vi "Agilent 3446X Series Acquire Multiple.vi"() -> ()   [LabVIEW 2021]
doc: "This example shows how to configure a measurement and take multiple readings."
uses:
  <instrlib>/Agilent 3446X Series/Public/Data/Read (Multiple Points).vi
  <instrlib>/Agilent 3446X Series/Agilent 3446X Series.lvlib
panel:
  in  "error in":errorcluster
  out "error out":errorcluster
  in  "Timeout(s)":i32=10000 format="%#.6g"
  in  "Sample Count":i32=1
  in  "Measurement Function":i32(ring)=10 items=["Continuity", "Current AC", "Current DC", "Diode", "Frequency", "Resistance 4-wire", "Period", "Resistance 2-wire", "Temperature", "Voltage AC", "Voltage DC", "Voltage DC Ratio", "Capacitance"]
  in  "Agilent DMM":refnum<visa-resource-name>
  out "Measurements":dbl[](array[numeric])
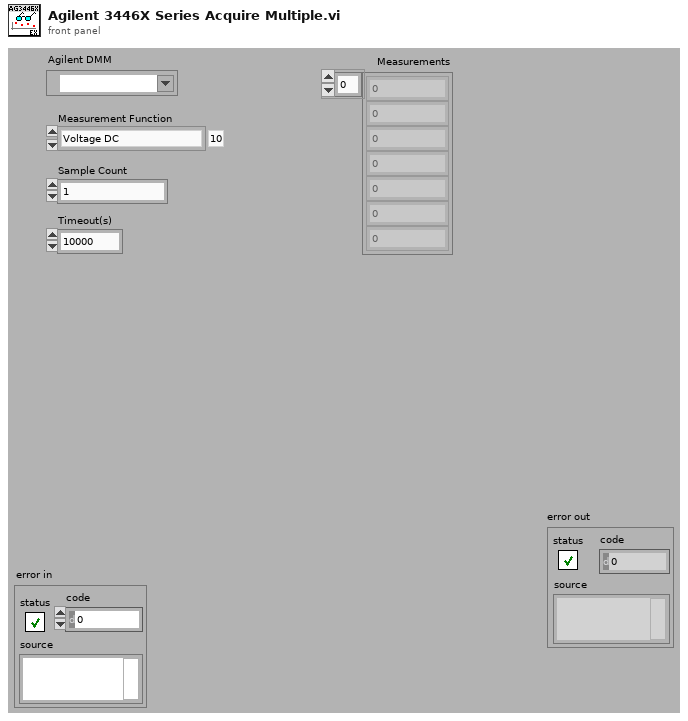
[diagram p1: front panel]
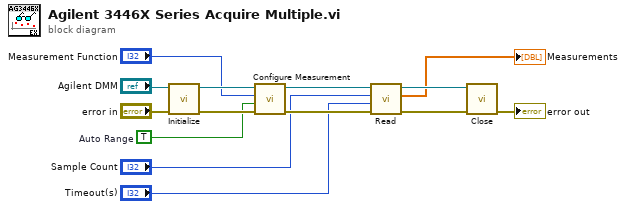
[diagram p0: block diagram]
diagram:
  w12 = TRUE  # Auto Range
  n1 = call <instrlib>:"Initialize.vi"("error in (no error)"="error in", "VISA resource name"="Agilent DMM") -> ("error out"=w13:errorcluster, "VISA resource name out"=w14:refnum<visa-resource-name>)  [unwired: 3 in, 5 out]
  n2 = call <instrlib>:"Configure Measurement.vi"("error in (no error)"=w13, "Auto Range (T: Enable)"=w12, "Measurement Function (10: Voltage DC)"="Measurement Function", "VISA resource name"=w14) -> ("error out"=w10:errorcluster, "VISA resource name out"=w9:refnum<visa-resource-name>)  [unwired: 2 in, 4 out]
  n3 = call-poly <instrlib>:"Read.vi"("error in (no error)"=w10, "Timeout (10000 ms)"="Timeout(s)", "Sample Count (1)"="Sample Count", "VISA resource name"=w9) -> ("error out"=w11:errorcluster, "Measurements"=→"Measurements":dbl[], "VISA resource name out"=w8:refnum<visa-resource-name>)  [unwired: 5 out]
  n4 = call <instrlib>:"Close.vi"("error in (no error)"=w11, "VISA resource name"=w8) -> ("error out"=→"error out":errorcluster)  [unwired: 9 out]
